vi "DELETE_snapshot_from_db.vi"(9 "SnapID":string, 10 "item":string, 11 "API Key":string="cheia04042025tema2restfulapi") -> (3 "DELETE_clear_specific_error_header":string)   [LabVIEW 2024]
uses:
  <vilib>/httpClient/LabVIEWHTTPClient.lvlib
panel:
  out "delete_error_":string
  out "error out delete error memory":errorcluster
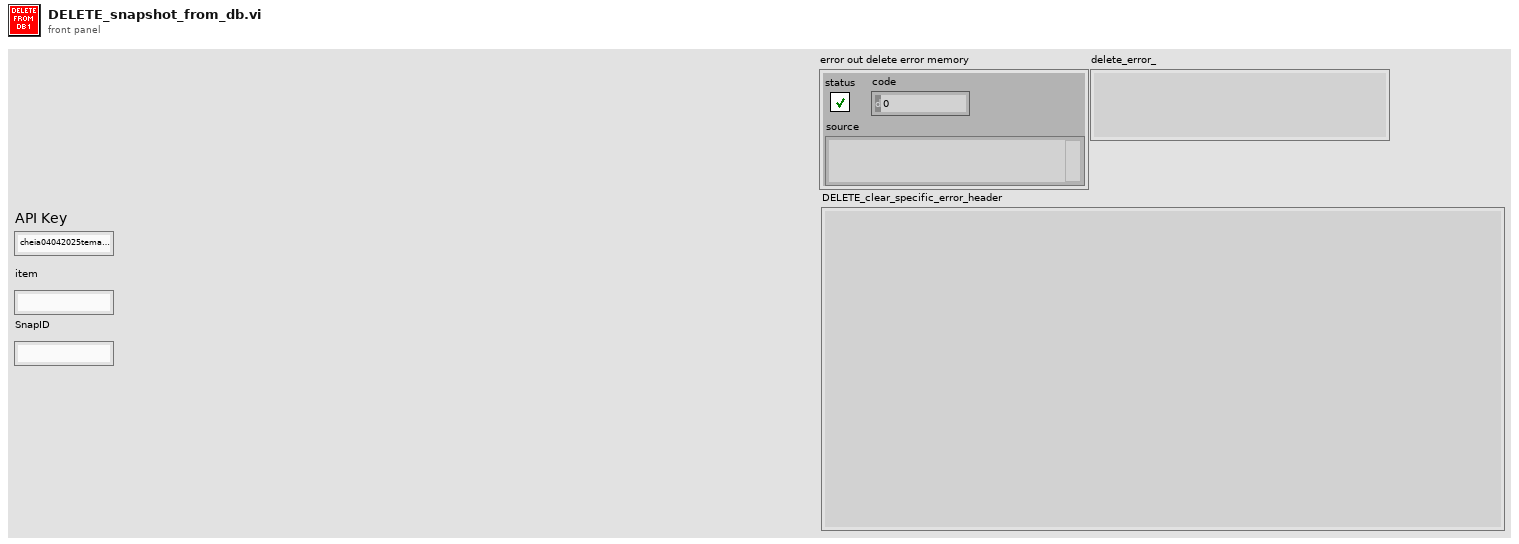
[diagram p1: front panel]
types:
  T1 = typedef "LabVIEWHTTPClient.lvlib/ClientHandle.ctl" = refnum<k1>
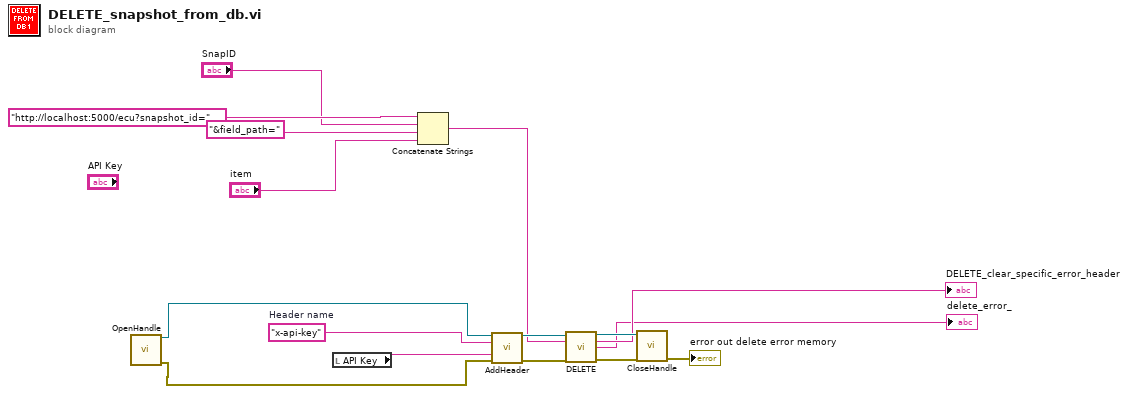
[diagram p0: block diagram]
diagram:
  w9 = "x-api-key"  # Header name
  n1 = call <vilib>:"OpenHandle.vi"() -> ("client handle out"=w10:T1, "error out"=w11:errorcluster)  [unwired: 14 in]
  n2 = local read "API Key"() -> (w8:string)
  n3 = Concatenate Strings("http://localhost:5000/ecu?snapshot_id=" ("url"), "SnapID", "&field_path=", "item") -> (w3:string)
  n4 = call <vilib>:"AddHeader.vi"("client handle"=w10, "header"=w9, "value"=w8, "error in (no error)"=w11) -> ("client handle out"=w13:T1, "error out"=w12:errorcluster)  [unwired: 10 in]
  n5 = call <vilib>:"DELETE.vi"("client handle"=w13, "url"=w3, "error in (no error)"=w12) -> ("client handle out"=w15:T1, "headers"=→"DELETE_clear_specific_error_header":string, "body"=→"delete_error_":string, "error out"=w14:errorcluster)  [unwired: 9 in]
  n6 = call <vilib>:"CloseHandle.vi"("client handle"=w15, "error in (no error)"=w14) -> ("error out"=→"error out delete error memory":errorcluster)  [unwired: 13 in]
